vi "Check next possible steps.vi"(10 "Indices":i32[](array[numeric])=[0], 11 "Array":cluster{i32[]}[](array[cluster])) -> (3 "output":dbl)   [LabVIEW 2018]
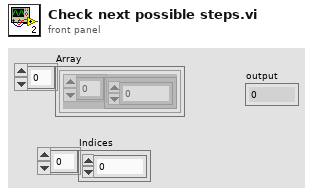
[diagram p1: front panel]
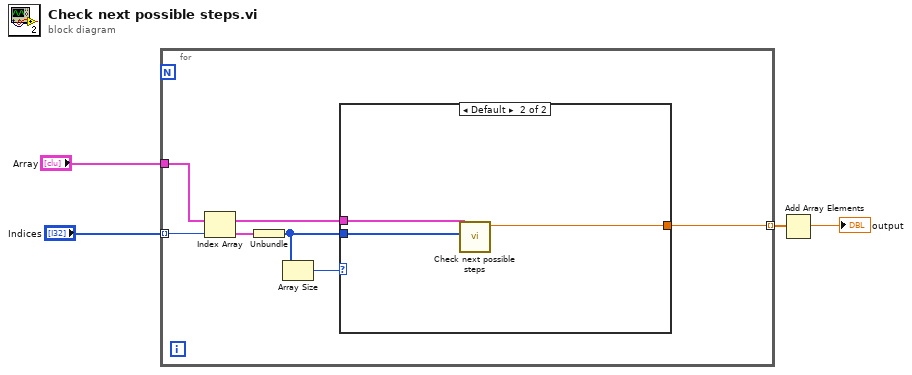
[diagram p0: block diagram]
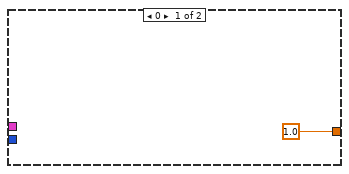
[diagram p2: hidden frame]
diagram:
  n1 = for {
    tunnel: "Array" -> [w7]
    tunnel: "Indices" -> [w6] mode=indexing
    tunnel: [w5] -> w1 mode=indexing
    n2 = Index Array(array=w7, index=w6) -> (element=w10:cluster{i32[]})
    n3 = Unbundle(w10) -> (w8:i32[])
    n4 = Array Size(array=w8) -> (size(s)=w9:i32)
    n5 = case shown="Default" w9 {
      tunnel: w8 -> [_ w14]
      tunnel: w7 -> [_ w13]
      tunnel: [1.0 w12] -> w5
      frame 0 {
      }
      frame Default {
        n6 = call "Check next possible steps.vi"("Indices"=w14, "Array"=w13) -> ("output"=w12:dbl)  [unwired: 9 in]
      }
    }
  }
  n7 = Add Array Elements(numeric array=w1) -> (sum=→"output":dbl)
